vi "1.6.1-CosDegIn_I-II.vi"(1 "theta":u8) -> (0 "Numeric":fxp<+/-,16,1> format="%.16g")   [LabVIEW 2010]
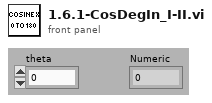
[diagram p1: front panel]
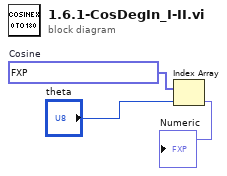
[diagram p0: block diagram]
diagram:
  w1 = fxp<+/-,16,1>[] [0.999969482421875, 0.999847412109375, 0.9993896484375, 0.998626708984375, 0.99755859375, 0.996185302734375, 0.9945068359375, 0.9925537109375, 0.990264892578125, 0.987701416015625, 0.98480224609375, 0.98162841796875, 0.9781494140625, 0.974365234375, 0.970306396484375, 0.965911865234375, 0.961273193359375, 0.956298828125, 0.9510498046875, 0.945526123046875, 0.939697265625, 0.93359375, 0.92718505859375, 0.920501708984375, 0.913543701171875, 0.90631103515625, 0.8988037109375, 0.891021728515625, 0.8829345703125, 0.8746337890625, 0.86602783203125, 0.857177734375, 0.848052978515625, 0.83868408203125, 0.82904052734375, 0.81915283203125, 0.80902099609375, 0.79864501953125, 0.78802490234375, 0.77716064453125, 0.76605224609375, 0.75469970703125, 0.743133544921875, 0.731353759765625, 0.719329833984375, 0.70709228515625, 0.694671630859375, 0.6820068359375, 0.66912841796875, 0.65606689453125, 0.642791748046875, 0.62933349609375, 0.61566162109375, 0.601806640625, 0.587799072265625, 0.573577880859375, 0.5592041015625, 0.544647216796875, 0.5299072265625, 0.515045166015625, 0.5, 0.48480224609375, 0.469482421875, 0.4539794921875, 0.438385009765625, 0.422607421875, 0.40673828125, 0.390716552734375, 0.374603271484375, 0.358367919921875, 0.342010498046875, 0.3255615234375, 0.30902099609375, 0.2923583984375, 0.275634765625, 0.258819580078125, 0.241912841796875, 0.224945068359375, 0.207916259765625, 0.1907958984375, 0.17364501953125, 0.15643310546875, 0.13916015625, 0.121856689453125, 0.104522705078125, 0.087158203125, 0.06976318359375, 0.052337646484375, 0.034912109375, 0.0174560546875, 0.0, -0.0174560546875, -0.034912109375, -0.052337646484375, -0.06976318359375, -0.087158203125, -0.104522705078125, -0.121856689453125, -0.13916015625, -0.15643310546875, -0.17364501953125, -0.1907958984375, -0.207916259765625, -0.224945068359375, -0.241912841796875, -0.258819580078125, -0.275634765625, -0.2923583984375, -0.30902099609375, -0.3255615234375, -0.342010498046875, -0.358367919921875, -0.374603271484375, -0.390716552734375, -0.40673828125, -0.422607421875, -0.438385009765625, -0.4539794921875, -0.469482421875, -0.48480224609375, -0.5, -0.515045166015625, -0.5299072265625, -0.544647216796875, -0.5592041015625, -0.573577880859375, -0.587799072265625, -0.601806640625, -0.61566162109375, -0.62933349609375, -0.642791748046875, -0.65606689453125, -0.66912841796875, -0.6820068359375, -0.694671630859375, -0.70709228515625, -0.719329833984375, -0.731353759765625, -0.743133544921875, -0.75469970703125, -0.76605224609375, -0.77716064453125, -0.78802490234375, -0.79864501953125, -0.80902099609375, -0.81915283203125, -0.82904052734375, -0.83868408203125, -0.848052978515625, -0.857177734375, -0.86602783203125, -0.8746337890625, -0.8829345703125, -0.891021728515625, -0.8988037109375, -0.90631103515625, -0.913543701171875, -0.920501708984375, -0.92718505859375, -0.93359375, -0.939697265625, -0.945526123046875, -0.9510498046875, -0.956298828125, -0.961273193359375, -0.965911865234375, -0.970306396484375, -0.974365234375, -0.9781494140625, -0.98162841796875, -0.98480224609375, -0.987701416015625, -0.990264892578125, -0.9925537109375, -0.9945068359375, -0.996185302734375, -0.99755859375, -0.998626708984375, -0.9993896484375, -0.999847412109375, -1.0]  # Cosine
  n1 = Index Array(array=w1, index="theta") -> (element=→"Numeric":fxp<+/-,16,1>)
